vi "ejemplo siso.vi"(11 "SP":dbl(slide) scale=0.0..360.0) -> (3 "Posicion":cluster{dbl, dbl}(knob)={0.0, 349.0774854239136})   [LabVIEW 2020]
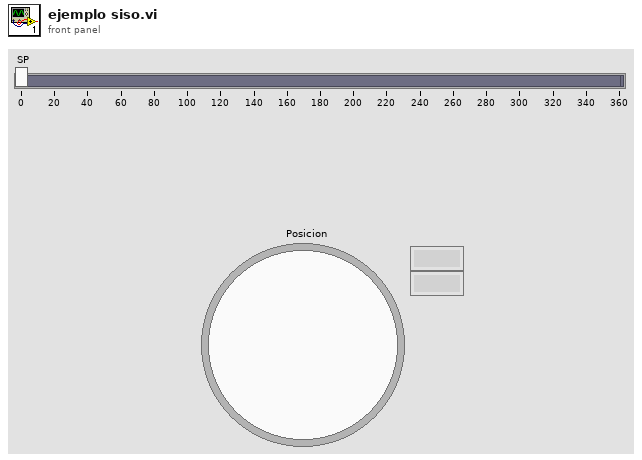
[diagram p1: front panel]
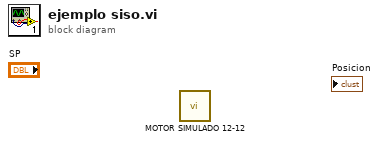
[diagram p0: block diagram]
diagram:
  n1 = call "MOTOR SIMULADO 12-12.vi"() -> ()  [unwired: 11 in, 1 out]
